vi "FindBlob_CenterOfMass.vi"(6 "Image in":T1 {"Dialogs" format="%.0b"}) -> (2 "center of mass Y":dbl[](array[numeric]), 3 "center of mass X":dbl[](array[numeric]))   [LabVIEW 2024]
uses:
  <userlib>/ImageProcessing/QTLIB_2595_LV86/QT_Image.ctl
panel:
  out "top":i32[](array[numeric])
  out "bottom":i32[](array[numeric])
  out "image":picture
  out "# particles":u32
  out "left":i32[](array[numeric])
  out "right":i32[](array[numeric])
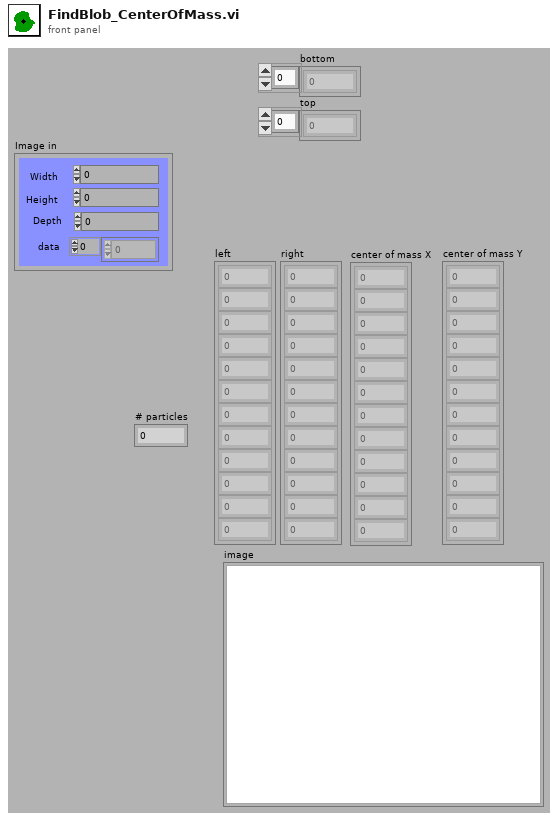
[diagram p1: front panel]
types:
  T1 = typedef "QT_Image.ctl" = cluster{"Width":i32, "Height":i32, "Depth":i32, "data":u8[], "Compressed data":u8[], "Color table":u32[], "Duration":i32, "Options":i32, "Timestamp":i32, "ID":i32, "Reserved":i32, "Dialogs":u32}
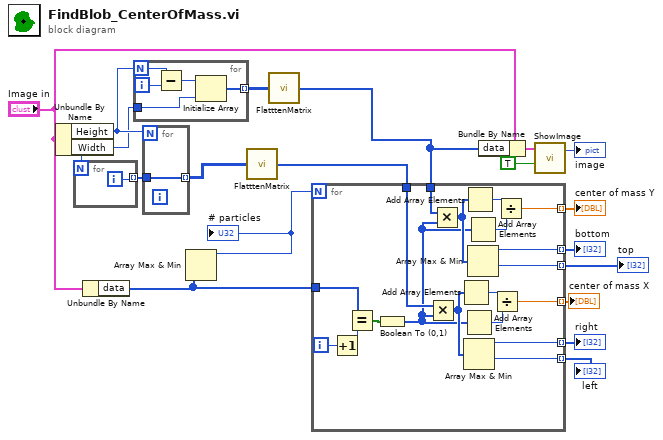
[diagram p0: block diagram]
diagram:
  n1 = Unbundle By Name("Image in") -> ("Height"=w5:i32, "Width"=w4:i32)
  n2 = for {
    N: w4 -> [_]
    tunnel: [w20] -> w19 mode=indexing
    i -> [w20]
  }
  n3 = Unbundle By Name("Image in") -> ("data"=w1:u8[])
  n4 = for {
    N: w5 -> [w23]
    tunnel: w4 -> [w25]
    tunnel: [w24] -> w3 mode=indexing
    i -> [w22]
    n5 = Subtract(x=w23, y=w22) -> (x-y=w21:i32)
    n6 = Initialize Array(w21, w25) -> (w24:i32[])
  }
  n7 = for {
    N: w5 -> [_]
    tunnel: w19 -> [w26]
    tunnel: [w26] -> w11 mode=indexing
  }
  n8 = Array Max & Min(array=w1) -> (max value=w10:u8)  [unwired: 3 out]
  "# particles" <- w10
  n9 = call <userlib>:"FlatttenMatrix.vi"("Matrix"=w11) -> ("Array"=w15:i32[])
  n10 = call <userlib>:"FlatttenMatrix.vi"("Matrix"=w3) -> ("Array"=w8:i32[])
  n11 = for {
    N: w10 -> [_]
    tunnel: w1 -> [w45]
    tunnel: w15 -> [w32]
    tunnel: [w41] -> w17 mode=indexing
    tunnel: [w40] -> w16 mode=indexing
    tunnel: [w36] -> w18 mode=indexing
    tunnel: w8 -> [w30]
    tunnel: [w29] -> w9 mode=indexing
    tunnel: [w28] -> w7 mode=indexing
    tunnel: [w27] -> w6 mode=indexing
    i -> [w44]
    n12 = Increment(x=w44) -> (x+1=w43:i32)
    n13 = Equal?(x=w45, y=w43) -> (x = y?=w42:bool[])
    n14 = Boolean To (0,1)(Boolean=w42) -> (0, 1=w31:i16[])
    n15 = Multiply(x=w32, y=w31) -> (x*y=w38:i32[])
    n16 = Multiply(x=w30, y=w31) -> (x*y=w34:i32[])
    n17 = Add Array Elements(numeric array=w38) -> (sum=w39:i32)
    n18 = Add Array Elements(numeric array=w31) -> (sum=w37:i16)
    n19 = Array Max & Min(array=w38) -> (max value=w41:i32, min value=w40:i32)  [unwired: 2 out]
    n20 = Add Array Elements(numeric array=w34) -> (sum=w33:i32)
    n21 = Add Array Elements(numeric array=w31) -> (sum=w35:i16)
    n22 = Array Max & Min(array=w34) -> (max value=w28:i32, min value=w27:i32)  [unwired: 2 out]
    n23 = Divide(x=w39, y=w37) -> (x/y=w36:dbl)
    n24 = Divide(x=w33, y=w35) -> (x/y=w29:dbl)
  }
  "center of mass X" <- w18
  "right" <- w17
  "left" <- w16
  "center of mass Y" <- w9
  "bottom" <- w7
  "top" <- w6
  n25 = Bundle By Name(cluster="Image in", "data"=w8) -> (w12:T1)
  n26 = call <userlib>:"ShowImage.vi"("Autoscale?"=TRUE, "Image"=w12) -> ("image"=→"image":picture)  [unwired: 1 in, 1 out]
